vi "标签.vi"(8 "错误输入（无错误）":errorcluster, 11 "引用":refnum<k24>) -> (0 "错误输出":errorcluster, 3 "引用输出":refnum<k24>)   [LabVIEW 2018]
uses:
  ScintillaNET.dll
  System.Drawing
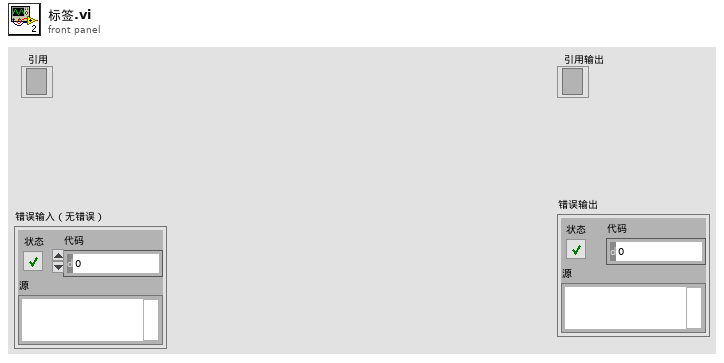
[diagram p1: front panel]
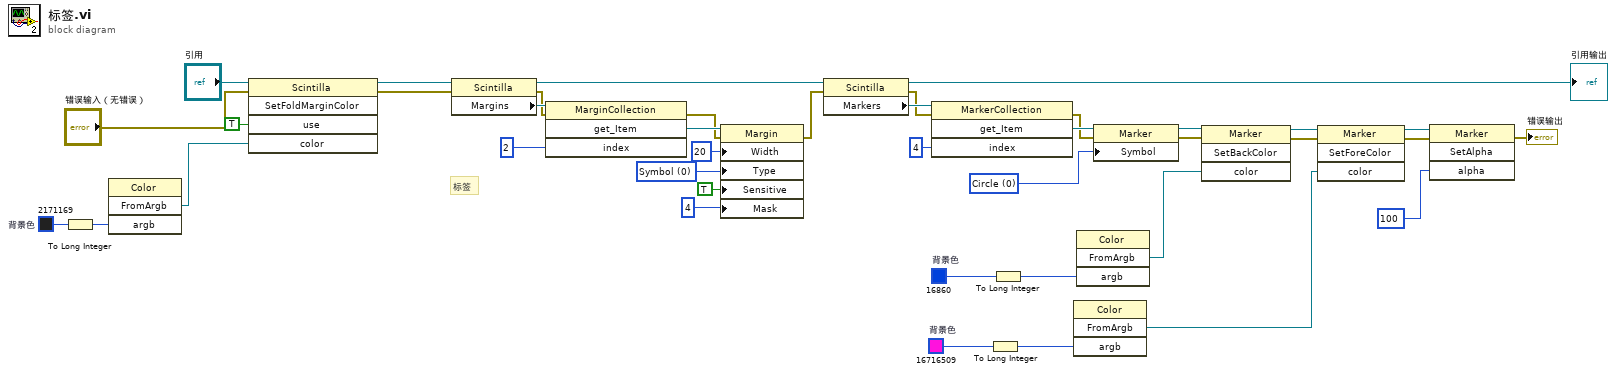
[diagram p0: block diagram]
diagram:
  w3 = u32 2171169  # 背景色
  w17 = u32 16716509  # 背景色
  w23 = u32 16860  # 背景色
  w27 = 0 items=["Circle"=0, "RoundRect"=1, "Arrow"=2, "SmallRect"=3, "ShortArrow"=4, "Empty"=5, "ArrowDown"=6, "Minus"=7, "Plus"=8, "VLine"=9, "LCorner"=10, "TCorner"=11, "BoxPlus"=12, "BoxPlusConnected"=13, "BoxMinus"=14, "BoxMinusConnected"=15, "LCornerCurve"=16, "TCornerCurve"=17, "CirclePlus"=18, "CirclePlusConnected"=19, "CircleMinus"=20, "CircleMinusConnected"=21, "Background"=22, "DotDotDot"=23, "Arrows"=24, "FullRect"=26, "LeftRect"=27, "Available"=28, "Underline"=29, "RgbaImage"=30, "Bookmark"=31] ("Symbol")
  w38 = 0 items=["Symbol", "Number", "BackColor", "ForeColor", "Text", "RightText", "Color"] ("Type")
  # "标签"
  n1 = To Long Integer(number=w3) -> (32bit integer=w2:i32)
  n2 = invoke class="Color" method="FromArgb"("argb"=w2) -> ("FromArgb"=w1:refnum<k24>)  [unwired: 3 in, 3 out]
  n3 = invoke on="调用节点" class="Scintilla" method="SetFoldMarginColor"(reference="引用", "use"=TRUE, "color"=w1) -> (reference out=w5:refnum<k24>)  [unwired: 2 in, 4 out]
  n4 = property class="Scintilla"(reference=w5, error in="错误输入（无错误）") -> (reference out=w32:refnum<k24>, error out=w15:errorcluster, "Margins"=w33:refnum<k24>)
  n5 = invoke class="MarginCollection" method="get_Item"(reference=w33, error in=w15, "index"=2) -> (error out=w14:errorcluster, "get_Item"=w35:refnum<k24>)  [unwired: 1 in, 2 out]
  n6 = property class="Margin"(reference=w35, error in=w14, "Width"=20, "Type"=w38, "Sensitive"=TRUE, "Mask"=u32 4) -> (error out=w13:errorcluster)  [unwired: 1 out]
  n7 = property class="Scintilla"(reference=w32, error in=w13) -> (reference out=→"引用输出":refnum<k24>, error out=w12:errorcluster, "Markers"=w31:refnum<k24>)
  n8 = invoke class="MarkerCollection" method="get_Item"(reference=w31, error in=w12, "index"=4) -> (error out=w11:errorcluster, "get_Item"=w29:refnum<k24>)  [unwired: 1 in, 2 out]
  n9 = To Long Integer(number=w17) -> (32bit integer=w18:i32)
  n10 = To Long Integer(number=w23) -> (32bit integer=w22:i32)
  n11 = invoke class="Color" method="FromArgb"("argb"=w18) -> ("FromArgb"=w16:refnum<k24>)  [unwired: 3 in, 3 out]
  n12 = invoke class="Color" method="FromArgb"("argb"=w22) -> ("FromArgb"=w21:refnum<k24>)  [unwired: 3 in, 3 out]
  n13 = property class="Marker"(reference=w29, error in=w11, "Symbol"=w27) -> (reference out=w28:refnum<k24>, error out=w10:errorcluster)
  n14 = invoke class="Marker" method="SetBackColor"(reference=w28, error in=w10, "color"=w21) -> (reference out=w26:refnum<k24>, error out=w9:errorcluster)  [unwired: 1 in, 2 out]
  n15 = invoke class="Marker" method="SetForeColor"(reference=w26, error in=w9, "color"=w16) -> (reference out=w25:refnum<k24>, error out=w8:errorcluster)  [unwired: 1 in, 2 out]
  n16 = invoke class="Marker" method="SetAlpha"(reference=w25, error in=w8, "alpha"=100) -> (error out=→"错误输出":errorcluster)  [unwired: 1 in, 3 out]
